vi "Change Speed Counter.vi"(8 "period(0.1s)":dbl=0.1 format="%#_13g", 11 "Numeric":dbl) -> (0 "New?":bool, 2 "Last Check Time":timestamp, 3 "Speed(#/s)":dbl)   [LabVIEW 2017, in "Communicable State Machine.lvlib"]
uses:
  Communicable State Machine.lvlib
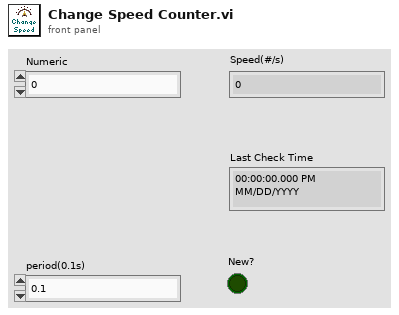
[diagram p1: front panel]
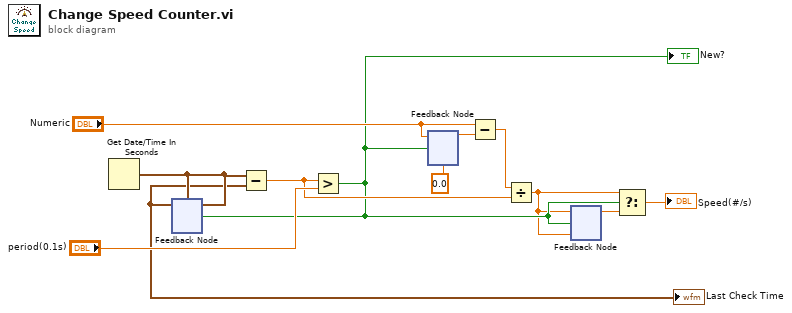
[diagram p0: block diagram]
diagram:
  n1 = Get Date/Time In Seconds() -> (seconds since 1Jan1904=w7:timestamp)
  n2 = feedback #1(w7) -> (w6:timestamp)
  "Last Check Time" <- w6
  n3 = Subtract(x=w7, y=w6) -> (x-y=w8:dbl)
  n4 = Greater?(x=w8, y="period(0.1s)") -> (0:w3:bool)
  "New?" <- w3
  n5 = feedback-in #1(w7, w3) -> ()
  n6 = feedback #2(0.0) -> (w12:dbl)
  n7 = feedback-in #2("Numeric", w3) -> ()
  n8 = Subtract(x="Numeric", y=w12) -> (x-y=w9:dbl)
  n9 = Divide(x=w9, y=w8) -> (x/y=w2:dbl)
  n10 = feedback #3(w2) -> (w4:dbl)
  n11 = feedback-in #3(w2, w3) -> ()
  n12 = Select(t=w2, s=w3, f=w4) -> (s? t:f=→"Speed(#/s)":dbl)
